vi "Is Null.vi"(1 "Port":refnum<class "FSM.Port.lvclass">) -> (0 "null":bool)   [LabVIEW 2020, in "FSM.Port.lvclass"]
uses:
  FSM.Port.lvclass
  FSM.Port.lvclass/FSM.Port.ctl
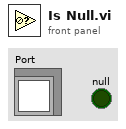
[diagram p1: front panel]
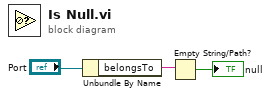
[diagram p0: block diagram]
diagram:
  n1 = Unbundle By Name("Port") -> ("belongsTo"=w2:string)
  n2 = Empty String/Path?(string/path=w2) -> (empty?=→"null":bool)
